vi "Return_Data.vi"(8 "error in (no error)":errorcluster caption="entrée d'erreur (pas d'erreur)", 11 "Class Instrument Multimeter en entrée":refnum<class "Class Instrument Balance.lvclass">) -> (0 "error out":errorcluster caption="sortie d'erreur", 2 "Data_Json":string, 3 "Class Instrument Multimeter en sortie":refnum<class "Class Instrument Balance.lvclass">)   [LabVIEW 2020, in "Library Instrument & Equipement.lvlib" / "Library Instruments.lvlib" / "Class Instrument Balance.lvclass"]
uses:
  Class Instrument Balance.lvclass
  Class Instrument Balance.lvclass/Class Instrument Balance.ctl
  JSON API/Variant JSON/Variant to JSON.vi
  JSON API/JSON Value/Get Item by name array.vi
  JSON API/JSON Value/JSON Value.lvclass
  JSON API/Get Polymorphic/JSON GetSet.lvlib
  JSON API/Variant JSON/Variant JSON.lvlib
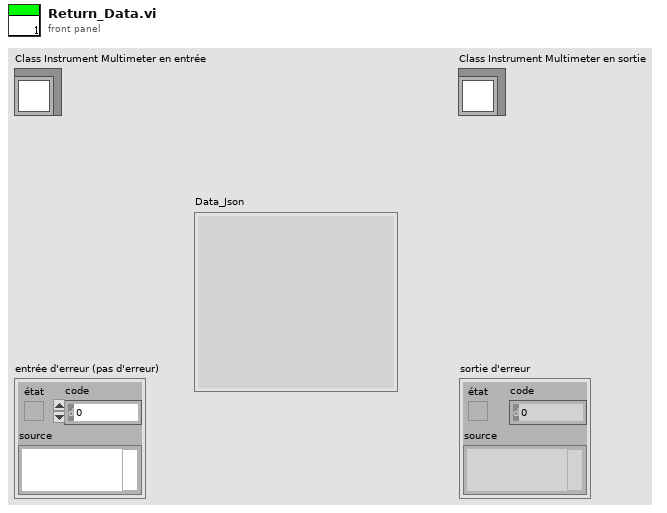
[diagram p1: front panel]
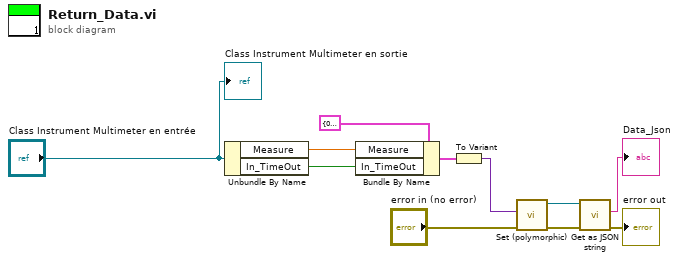
[diagram p0: block diagram]
diagram:
  n1 = Unbundle By Name("Class Instrument Multimeter en entrée") -> ("Measure"=w2:dbl, "In_TimeOut"=w1:bool)
  n2 = Bundle By Name(cluster=cluster{"Measure":dbl, "In_TimeOut":bool} {"Measure"=0.0, "In_TimeOut"=FALSE}, "Measure"=w2, "In_TimeOut"=w1) -> (w3:cluster{"Measure":dbl, "In_TimeOut":bool})
  n3 = To Variant(anything=w3) -> (Variant=w6:variant)
  n4 = call-poly "Set (polymorphic).vi"("error in (no error)"="error in (no error)", "Variant"=w6) -> ("error out"=w10:errorcluster, "JSON Value out"=w11:refnum<class "JSON Value.lvclass">)  [unwired: 8 in]
  n5 = call "Get as JSON string.vi"("error in (no error)"=w10, "JSON Value in"=w11) -> ("error out"=→"error out":errorcluster, "<JSON>"=→"Data_Json":string)  [unwired: 8 in]
  "Class Instrument Multimeter en sortie" <- "Class Instrument Multimeter en entrée"
